vi "V104 VISA to Host (SubVI).vi"(7 "Serial Queue In":refnum<queue>, 8 "error in (no error)":errorcluster, 10 "Serial Settings":T1={"baud rate"=9600, "data bits"=8, "parity"=enum."None", "stop bits"=10, "flow control"=0} {"flow control" items=["None"=0, "XON/XOFF"=1, "RTS/CTS"=2, "DTR/DSR"=4]; "stop bits" items=["1.0"=10, "1.5"=15, "2.0"=20]; "data bits" min=5 max=8 step=1; "baud rate" items=["75"=75, "110"=110, "134"=134, "150"=150, "300"=300, "600"=600, "1200"=1200, "1800"=1800, "2400"=2400, "4800"=4800, "7200"=7200, "9600"=9600, "14400"=14400, "19200"=19200, "28800"=28800, "38400"=38400, "56000"=56000, "57600"=57600, "115200"=115200, "128000"=128000, "230400"=230400]}, 11 "VISA resource name":refnum<visa-resource-name>="COM1") -> (0 "error out":errorcluster)   [LabVIEW 2019]
doc: "This SubVI interacts with the FPGA code to read measurement data from a DMA FIFO. It waits for the FPGA to assert an interrupt, signalling that a data packet is ready to be read. It then reads that FIFO and sends the FPGA an IRQ acknowlegement. It rebuilds the data packet header with bytes that were *consumed* as part of the FPGA stream screening process. This rebuild is necessary for the checksum process to work. Data are output to a Stream Chennel. \n\n2020 NREL"
uses:
  Globals and Definitions/Serial - Settings.ctl
  <vilib>/Instr/_visa.llb/VISA Configure Serial Port (Instr).vi
  Globals and Definitions/RT Globals RD v1.0.vi
panel:
  in  "Read Count":u32=1000
  in  "Termination Character":u8=10 format="%.0x"
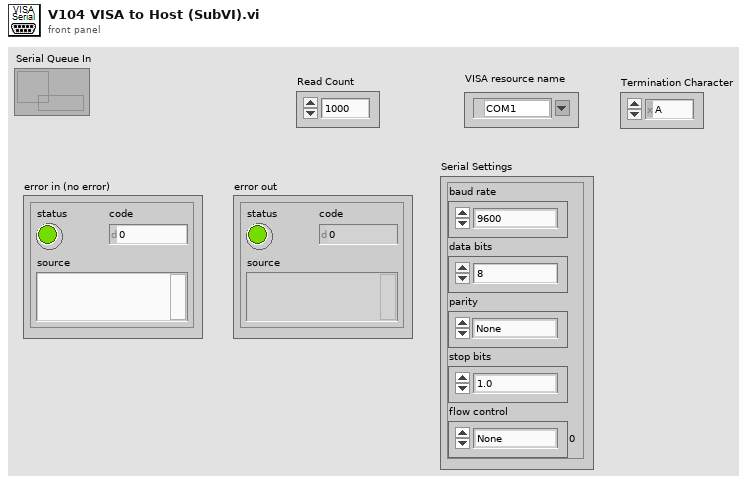
[diagram p1: front panel]
types:
  T1 = typedef "Serial - Settings.ctl" = cluster{"baud rate":u32, "data bits":u16, "parity":enum16{"None", "Odd", "Even", "Mark", "Space"}, "stop bits":u16, "flow control":u16}
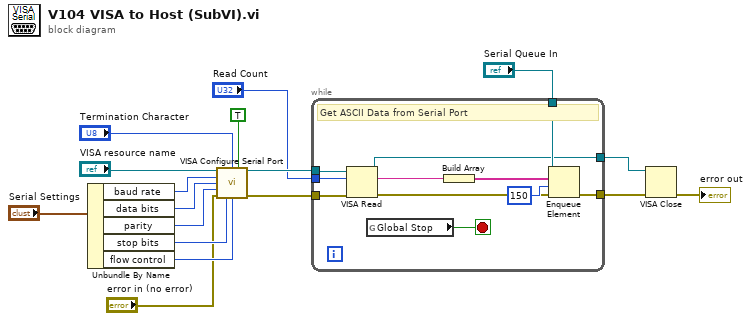
[diagram p0: block diagram]
diagram:
  n1 = Unbundle By Name("Serial Settings") -> ("baud rate"=w10:u32, "data bits"=w11:u16, "parity"=w12:enum16{"None", "Odd", "Even", "Mark", "Space"}, "stop bits"=w13:u16, "flow control"=w17:u16)
  n2 = call-poly "VISA Configure Serial Port"("VISA resource name"="VISA resource name", "termination char\n(0xA = '\\n' = LF)"="Termination Character", "Enable Termination\nChar (T)"=TRUE ("Enable Termination\nChar (T)"), "baud rate (9600)"=w10, "data bits (8)"=w11, "parity (0:none)"=w12, "error in (no error)"="error in (no error)", "stop bits (10: 1 bit)"=w13, "flow control (0:none)"=w17) -> ("VISA resource name out"=w7:refnum<visa-resource-name>, "error out"=w6:errorcluster)  [unwired: 1 in, 4 out]
  n3 = while {
    tunnel: "Serial Queue In" -> [w27]
    tunnel: w6 -> [w24]
    tunnel: w7 -> [w25]
    tunnel: [w22] -> w5
    tunnel: [w21] -> w4
    tunnel: "Read Count" -> [w20]
    stop <- w28 stop-if-true
    # "Get ASCII Data from Serial Port"
    n4 = VISA Read(VISA resource name=w25, byte count=w20, error in (no error)=w24) -> (VISA resource name out=w22:refnum<visa-resource-name>, read buffer=w19:string, error out=w23:errorcluster)  [unwired: 1 out]
    n5 = global read "RT Globals RD v1.0.vi" "Global Stop"() -> (w28:bool)
    n6 = Build Array(w19) -> (w18:string[])
    n7 = Enqueue Element(queue=w27, element=w18, timeout in ms (-1)=150, error in (no error)=w23) -> (error out=w21:errorcluster)  [unwired: 2 out]
  }
  n8 = VISA Close(VISA resource name=w5, error in (no error)=w4) -> (error out=→"error out":errorcluster)
